vi "Set Fixed Emissivity.vi"(10 "Value":sgl, 11 "index":u16) -> (3 "function return":sgl)   [LabVIEW 2025, in "ExtremelyEpicImagerIPC2.lvlib"]
doc: "IMAGERIPC_API float WINAPI SetFixedEmissivity(WORD index, float Value);"
uses:
  ExtremelyEpicImagerIPC2.lvlib
  ImagerIPC2.dll
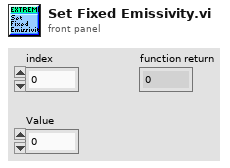
[diagram p1: front panel]
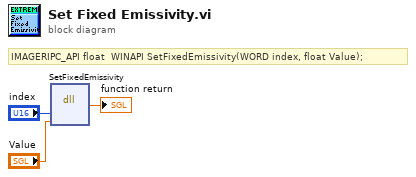
[diagram p0: block diagram]
diagram:
  # "IMAGERIPC_API float\t WINAPI SetFixedEmissivity(WORD index, float Value);"
  n1 = dll-call lib="C:/Users/mayhe/OneDrive/Documents/GitHub/In-situ-monitoring-of-powder-bed-fusion-additive-manufacturing/system_development/Orichalcum/v0.2/Software_design/thermal-camera/VI/Connect SDK/ImagerIPC2.*" fn="SetFixedEmissivity"("index"="index", "Value"="Value") -> (→"function return":sgl)  [unwired: 5 in, 2 out]
